vi "LogFileOpened Event Callback.vi"(4 "File Opened Event":refnum<user-event>, 5 "Event Data":cluster{"sender":refnum<k24>, "e":refnum<k24>}, 6 "Data Logging Manager Ref":T1, 7 "Event Common Data":T2) -> ()   [LabVIEW 2020, in "NI_VS Data Logging API.lvlib"]
uses:
  <vilib>/NI VeriStand/Execution/DataLogging/NI_VS Data Logging API.lvlib
  <vilib>/NI VeriStand/Execution/DataLogging/IDataLogging Ref.ctl
  NationalInstruments.VeriStand.ClientAPI
  <vilib>/NI VeriStand/Execution/DataLogging/Log File Opened Event Data.ctl
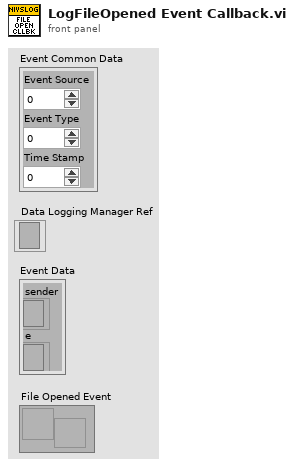
[diagram p1: front panel]
types:
  T1 = typedef "NI_VS Data Logging API.lvlib/IDataLogging Ref.ctl" = refnum<k24>
  T2 = cluster{"Event Source":i32, "Event Type":u32, "Time Stamp":u32}
  T3 = typedef "NI_VS Data Logging API.lvlib/Log File Opened Event Data.ctl" = cluster{"Session Name":string, "Log File Path":path}
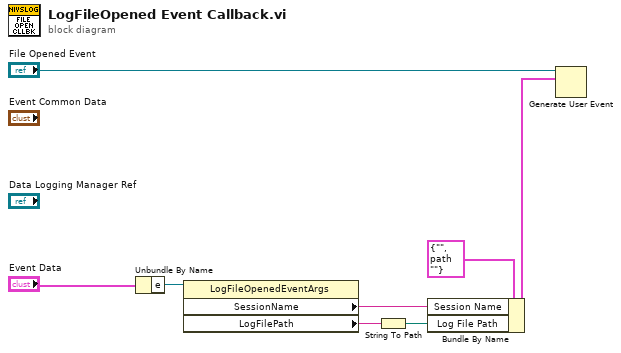
[diagram p0: block diagram]
diagram:
  n1 = Unbundle By Name("Event Data") -> ("e"=w4:refnum<k24>)
  n2 = property class="LogFileOpenedEventArgs"(reference=w4) -> ("SessionName"=w3:string, "LogFilePath"=w2:string)  [unwired: 1 in, 2 out]
  n3 = String To Path(string=w2) -> (path=w1:path)
  n4 = Bundle By Name(cluster=T3 {"Session Name"="", "Log File Path"=path ""} ("event data"), "Session Name"=w3, "Log File Path"=w1) -> (w6:T3)
  n5 = Generate User Event(user event="File Opened Event", event data cluster=w6) -> ()  [unwired: 2 in, 2 out]
